vi "FindPosForItem.vi"(0 "reference":refnum<class "ClassNode.lvclass">, 1 "SearchItem":string, 2 "AttributesIDs":string[](array[string]), 3 "MethodIDs":string[](array[string]), 5 "error in (no error)":errorcluster) -> (12 "UpperRightPoint":T1 {"y" format="%.2f"; "x" format="%.2f"}, 14 "reference out":refnum<class "ClassNode.lvclass">, 15 "LeftPoint":T1 {"y" format="%.2f"; "x" format="%.2f"}, 16 "CenterPoint":T1 {"y" format="%.2f"; "x" format="%.2f"}, 17 "RightPoint":T1 {"y" format="%.2f"; "x" format="%.2f"}, 18 "UpperLeftPoint":T1 {"y" format="%.2f"; "x" format="%.2f"}, 19 "error out":errorcluster)   [LabVIEW 2014, in "ClassNode.lvclass"]
doc: "public void draw(Graphics2D g2, Point2D p, Point2D q)"
uses:
  <resource>/Framework/Providers/Open_GDS/UML/ClassNode_class/ClassNode.lvclass
  <resource>/Framework/Providers/Open_GDS/UML/General/Point/Point Point2D.ctl
  <resource>/Framework/Providers/Open_GDS/UML/General/Rectangle/Rectangle Rectangle2D.ctl
  <resource>/Framework/Providers/Open_GDS/UML/MultiLineString_class/MultiLineString.lvclass
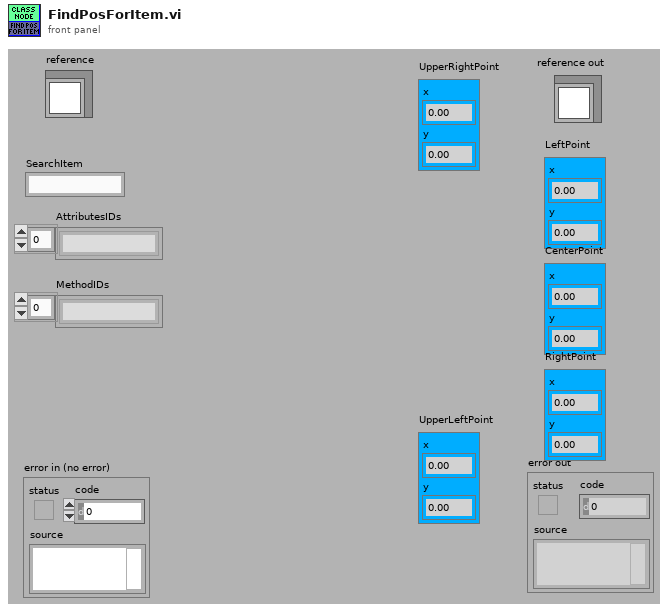
[diagram p1: front panel]
types:
  T1 = typedef "Point Point2D.ctl" = cluster{"x":dbl, "y":dbl}
  T2 = typedef "Rectangle Rectangle2D.ctl" = cluster{"x":dbl, "y":dbl, "width":dbl, "height":dbl}
  T3 = typedef "ClassNode.lvclass/ObjectAttributes.ctl" = cluster{"Base class":T4, "midHeight":dbl, "botHeight":dbl, "name":refnum<class "MultiLineString.lvclass">, "attributes":refnum<class "MultiLineString.lvclass">, "methods":refnum<class "MultiLineString.lvclass">, "DEFAULT_COMPARTMENT_HEIGHT":i32, "DEFAULT_WIDTH":i32, "DEFAULT_HEIGHT":i32, "showMethods":bool, "showAttributes":bool, "ClassPath":path}
  T4 = typedef "RectangularNode.lvclass/ObjectAttributes.ctl" = cluster{"Base class":T5, "bounds":T2}
  T5 = typedef "AbstractNode.lvclass/ObjectAttributes.ctl" = cluster{"parent":refnum<class "AbstractNode.lvclass">, "children":refnum<class "AbstractNode.lvclass">[], "Hidden":bool}
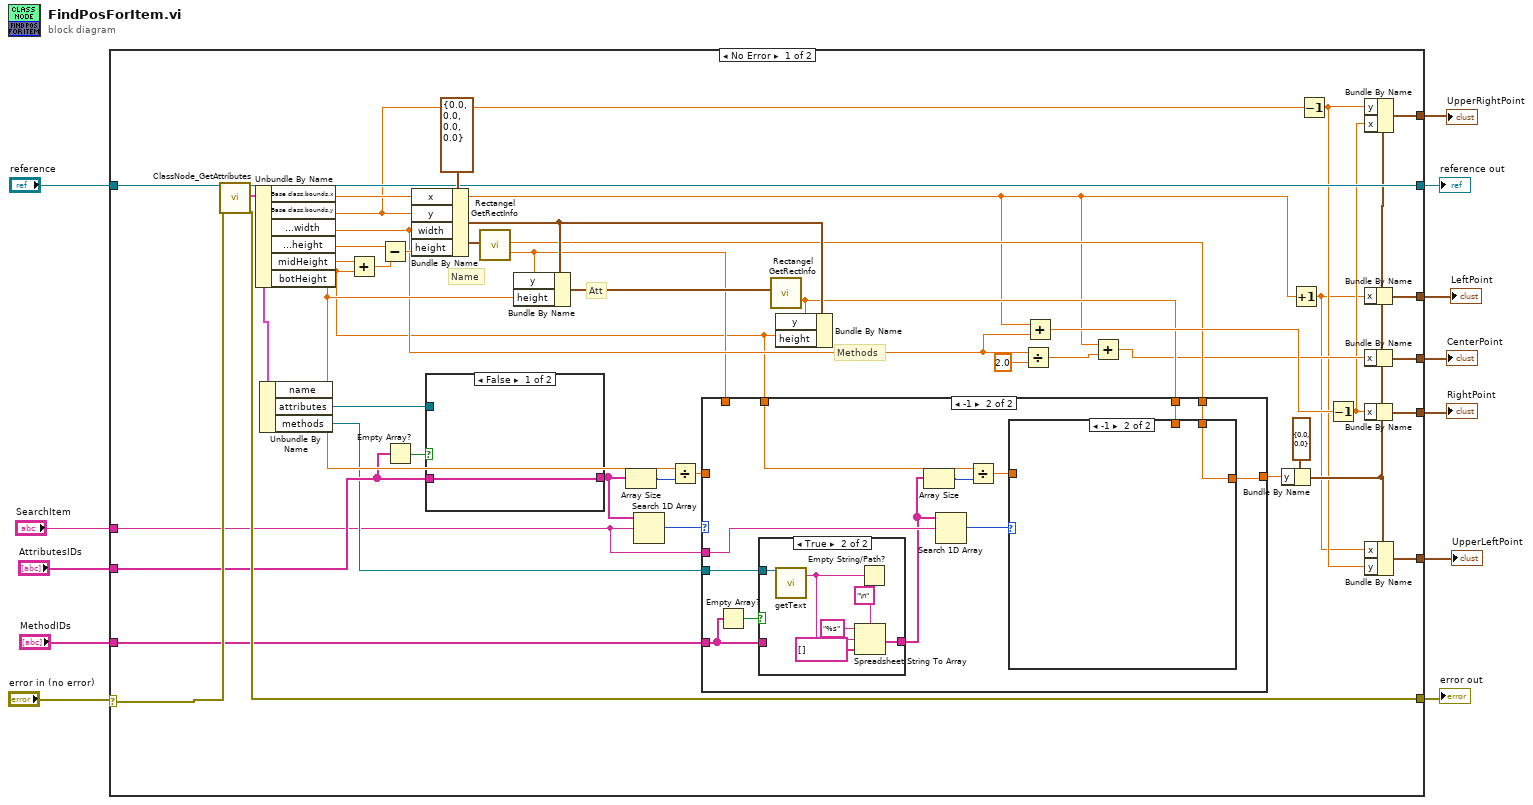
[diagram p0: block diagram]
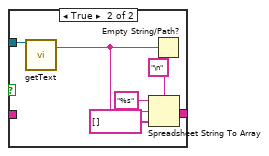
[diagram p2: hidden frame]
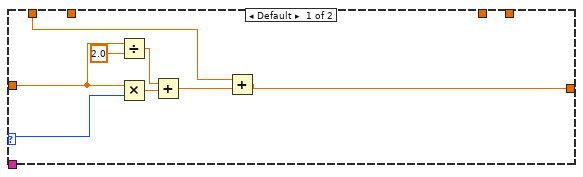
[diagram p3: hidden frame]
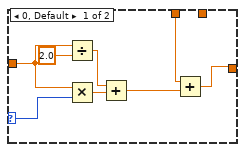
[diagram p4: hidden frame]
diagram:
  n1 = case shown="No Error" "error in (no error)" {
    selector: "error in (no error)" -> [w55 w100]
    tunnel: "reference" -> [w56 w101]
    tunnel: [w44 w100] -> w11
    tunnel: [w49 w101] -> w10
    tunnel: "SearchItem" -> [w27 _]
    tunnel: "AttributesIDs" -> [w38 _]
    tunnel: [w35 _] -> w6
    tunnel: [w33 _] -> w5
    tunnel: [w32 _] -> w4
    tunnel: "MethodIDs" -> [w29 _]
    tunnel: [w17 _] -> w2
    tunnel: [w15 _] -> w1
    frame No Error {
      # "Methods"
      # "Att"
      # "Name"
      n2 = call <resource>:"ClassNode_GetAttributes.vi"("reference in"=w56, "error in (no error)"=w55) -> ("reference out"=w49:refnum<class "ClassNode.lvclass">, "Attributes"=w54:T3, "error out"=w44:errorcluster)  [unwired: 15 out]
      n3 = Unbundle By Name(w54) -> ("Base class.bounds.x"=w22:dbl, "Base class.bounds.y"=w18:dbl, "Base class.bounds.width"=w31:dbl, "Base class.bounds.height"=w52:dbl, "midHeight"=w42:dbl, "botHeight"=w23:dbl)
      n4 = Unbundle By Name(w54) -> ("attributes"=w45:refnum<class "MultiLineString.lvclass">, "methods"=w28:refnum<class "MultiLineString.lvclass">)  [unwired: 1 out]
      n5 = Add(x=w42, y=w23) -> (x+y=w50:dbl)
      n6 = Subtract(x=w52, y=w50) -> (x-y=w51:dbl)
      n7 = Empty Array?(array=w38) -> (empty?=w39:bool)
      n8 = Bundle By Name(cluster=T2 {"x"=0.0, "y"=0.0, "width"=0.0, "height"=0.0} ("points"), "x"=w22, "y"=w18, "width"=w31, "height"=w51) -> (w48:T2)
      n9 = case shown="False" w39 {
        tunnel: [w57 w59] -> w46
        tunnel: w45 -> [_ w58]
        tunnel: w38 -> [w57 _]
        frame False {
        }
        frame True {
          n10 = call-dynamic "getText.vi"("reference"=w58) -> ("text"=w60:string)  [unwired: 1 in, 17 out]
          n11 = Spreadsheet String To Array(delimiter (Tab)="\n", format string="%s", spreadsheet string=w60, array type (2D Dbl)=string[] []) -> (array=w59:string[])
          n12 = Empty String/Path?(string/path=w60) -> ()  [unwired: 1 out]
        }
      }
      n13 = call <resource>:"Rectangel GetRectInfo.vi"("bounds"=w48) -> ("centerY"=w25:dbl, "maxY"=w26:dbl)  [unwired: 1 in, 16 out]
      n14 = Bundle By Name(cluster=w48, "y"=w26, "height"=w42) -> (w47:T2)
      n15 = Array Size(array=w46) -> (size(s)=w43:i32)
      n16 = Search 1D Array(1D array=w46, element=w27) -> (index of element=w40:i32)  [unwired: 1 in]
      n17 = Divide(x=w42, y=w43) -> (x/y=w41:dbl)
      n18 = call <resource>:"Rectangel GetRectInfo.vi"("bounds"=w47) -> ("maxY"=w24:dbl)  [unwired: 1 in, 17 out]
      n19 = case shown="-1" w40 {
        selector: w40 -> [w71 _]
        tunnel: w41 -> [w69 _]
        tunnel: [w64 w75] -> w36
        tunnel: w29 -> [_ w82]
        tunnel: w28 -> [_ w81]
        tunnel: w27 -> [_ w79]
        tunnel: w26 -> [w65 _]
        tunnel: w25 -> [_ w76]
        tunnel: w24 -> [_ w74]
        tunnel: w23 -> [_ w73]
        frame Default {
          n20 = Divide(x=w69, y=2.0) -> (x/y=w67:dbl)
          n21 = Multiply(x=w69, y=w71) -> (x*y=w70:dbl)
          n22 = Add(x=w67, y=w70) -> (x+y=w66:dbl)
          n23 = Add(x=w65, y=w66) -> (x+y=w64:dbl)
        }
        frame -1 {
          n24 = Empty Array?(array=w82) -> (empty?=w83:bool)
          n25 = case shown="True" w83 {
            tunnel: [w93 w95] -> w78
            tunnel: w81 -> [_ w94]
            tunnel: w82 -> [w93 _]
            frame False {
            }
            frame True {
              n26 = call-dynamic "getText.vi"("reference"=w94) -> ("text"=w96:string)  [unwired: 1 in, 17 out]
              n27 = Spreadsheet String To Array(delimiter (Tab)="\n", format string="%s", spreadsheet string=w96, array type (2D Dbl)=string[] []) -> (array=w95:string[])
              n28 = Empty String/Path?(string/path=w96) -> ()  [unwired: 1 out]
            }
          }
          n29 = Array Size(array=w78) -> (size(s)=w80:i32)
          n30 = Search 1D Array(1D array=w78, element=w79) -> (index of element=w77:i32)  [unwired: 1 in]
          n31 = Divide(x=w73, y=w80) -> (x/y=w72:dbl)
          n32 = case shown="-1" w77 {
            selector: w77 -> [w84 _]
            tunnel: w76 -> [_ w92]
            tunnel: [w86 w92] -> w75
            tunnel: w74 -> [w87 _]
            tunnel: w72 -> [w85 _]
            frame 0, Default {
              n33 = Divide(x=w85, y=2.0) -> (x/y=w89:dbl)
              n34 = Multiply(x=w85, y=w84) -> (x*y=w91:dbl)
              n35 = Add(x=w89, y=w91) -> (x+y=w88:dbl)
              n36 = Add(x=w87, y=w88) -> (x+y=w86:dbl)
            }
            frame -1 {
            }
          }
        }
      }
      n37 = Bundle By Name(cluster=w48, "y"=w24, "height"=w23) -> ()  [unwired: 1 out]
      n38 = Divide(x=w31, y=2.0) -> (x/y=w21:dbl)
      n39 = Add(x=w22, y=w31) -> (x+y=w30:dbl)
      n40 = Add(x=w22, y=w21) -> (x+y=w20:dbl)
      n41 = Bundle By Name(cluster=T1 {"x"=0.0, "y"=0.0} ("LeftPoint"), "y"=w36) -> (w16:T1)
      n42 = Increment(x=w22) -> (x+1=w13:dbl)
      n43 = Decrement(x=w18) -> (x-1=w14:dbl)
      n44 = Decrement(x=w30) -> (x-1=w19:dbl)
      n45 = Bundle By Name(cluster=w16, "y"=w14, "x"=w19) -> (w17:T1)
      n46 = Bundle By Name(cluster=w16, "x"=w13) -> (w35:T1)
      n47 = Bundle By Name(cluster=w16, "x"=w20) -> (w33:T1)
      n48 = Bundle By Name(cluster=w16, "x"=w19) -> (w32:T1)
      n49 = Bundle By Name(cluster=w16, "x"=w13, "y"=w14) -> (w15:T1)
    }
    frame Error {
    }
  }
  "reference out" <- w10
  "error out" <- w11
  "LeftPoint" <- w6
  "CenterPoint" <- w5
  "RightPoint" <- w4
  "UpperRightPoint" <- w2
  "UpperLeftPoint" <- w1
